vi "remove input channels which dont have a pair.vi"(7 "instance id":string, 8 "output channels":refnum<class "TBM channel.lvclass">[](array[class]), 9 "input channels":refnum<class "TBM channel.lvclass">[](array[class]), 10 "engine configuration in":refnum<class "engine configuration.lvclass">, 11 "TEC configuration in":refnum<class "TEC configuration.lvclass">) -> (1 "input channels out":refnum<class "TBM channel.lvclass">[](array[class]), 2 "engine configuration out":refnum<class "engine configuration.lvclass">, 3 "TEC configuration out":refnum<class "TEC configuration.lvclass">)   [LabVIEW 2013, in "TEC editor node.lvclass"]
uses:
  TEC editor node.lvclass
  configuration/TEC configuration.lvclass
  <vilib>/NI/Module Execution Interface/Engine Configuration/engine configuration.lvclass
  <vilib>/NI/Tag Bus Module Framework/channel/TBM channel.lvclass
  <vilib>/NI/Tag Bus/tag/tag descriptor.lvclass/tag descriptor.ctl
  <vilib>/NI/Tag Bus/tag/tag descriptor.lvclass
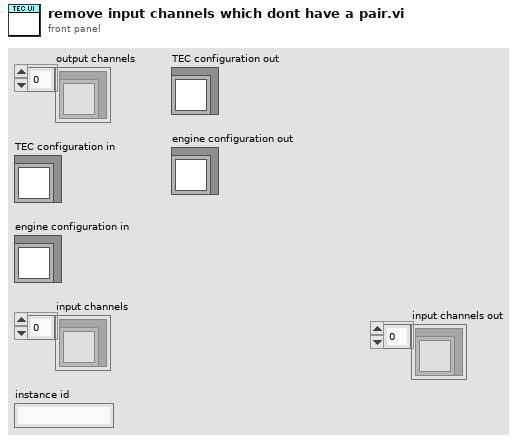
[diagram p1: front panel]
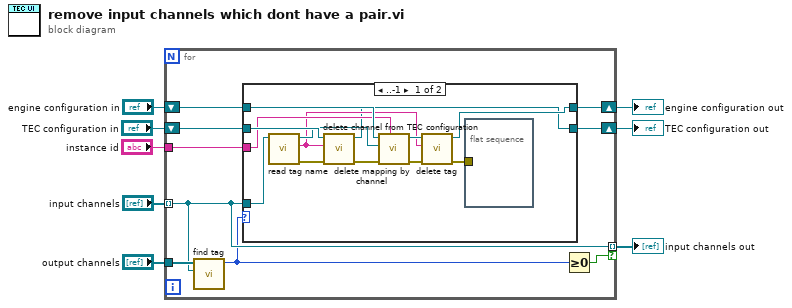
[diagram p0: block diagram]
diagram:
  n1 = for {
    shift-right: [w14] -> w7
    shift-left: "engine configuration in" -> [w16]
    shift-right: [w13] -> w8
    shift-left: "TEC configuration in" -> [w15]
    tunnel: "input channels" -> [w11] mode=indexing
    tunnel: "output channels" -> [w17]
    tunnel: "instance id" -> [w12]
    tunnel: [w11] -> w1 mode=indexing if=w9
    n2 = call <vilib>:"find tag.vi"("tag"=w11, "tags in"=w17) -> ("index"=w10:i32)  [unwired: 9 in]
    n3 = case shown="..-1" w10 {
      tunnel: w16 -> [w26 w32]
      tunnel: w15 -> [w30 w31]
      tunnel: [w20 w32] -> w14
      tunnel: [w19 w31] -> w13
      tunnel: w11 -> [w29 _]
      tunnel: w12 -> [w24 _]
      frame ..-1 {
        n4 = call <vilib>:"read tag name.vi"("system tag in"=w29) -> ("error out"=w28:errorcluster, "name"=w21:string, "system tag out"=w25:refnum<class "TBM channel.lvclass">)  [unwired: 8 in]
        n5 = call "delete channel from TEC configuration.vi"("error in"=w28, "channel to delete"=w21, "TEC configuration in"=w30) -> ("error out"=w27:errorcluster, "TEC configuration out"=w19:refnum<class "TEC configuration.lvclass">)  [unwired: 7 in]
        n6 = call <vilib>:"delete mapping by channel.vi"("owner ID"=w24, "error in"=w27, "channel"=w25, "engine configuration in"=w26) -> ("error out"=w22:errorcluster, "engine configuration out"=w23:refnum<class "engine configuration.lvclass">)  [unwired: 6 in]
        n7 = call <vilib>:"delete tag.vi"("error in"=w22, "tag name"=w21, "engine configuration in"=w23) -> ("error out"=w18:errorcluster, "engine configuration out"=w20:refnum<class "engine configuration.lvclass">)  [unwired: 7 in]
        n8 = flat-sequence {
          tunnel: w18 -> [_]
          frame #0 {
          }
        }
      }
      frame 0.. {
        # "ok"
      }
    }
    n9 = Greater Or Equal To 0?(x=w10) -> (x >= 0?=w9:bool)
  }
  "TEC configuration out" <- w8
  "engine configuration out" <- w7
  "input channels out" <- w1
